vi "test_serialize_deserialize.vi"   [LabVIEW 2020, in "GPS.lvlib"]
doc: "Version 0.1"
uses:
  <vilib>/ADAS Record/CustomDataTypes/GPS/GPS.lvlib
  <vilib>/addons/_JKI Toolkits/Caraya/classes/Test/Test.lvclass
  <vilib>/addons/_JKI Toolkits/Caraya/classes/Assert/Assert.lvclass
  <vilib>/ADAS Record/CustomDataTypes/GPS/Process Data.ctl
  <vilib>/ADAS Record/CustomDataTypes/GPS/Serialize Data.vi
  <vilib>/ADAS Record/CustomDataTypes/GPS/Deserialize Data.vi
types:
  T1 = cluster{"Latitude":dbl, "Longitude":dbl, "Altitude":dbl}
  T2 = typedef "GPS.lvlib/Process Data.ctl" = cluster{"Timestamp":u64, "Antenna Connected":bool, "Satellites":u32, "Mobile Mode":bool, "Location":cluster{"Latitude":dbl, "Longitude":dbl, "Altitude":dbl}, "Velocity":cluster{"East":dbl, "North":dbl, "Up":dbl}, "GPS state":u32, "UTC Offset":i32, "UTC Offset Valid":bool}
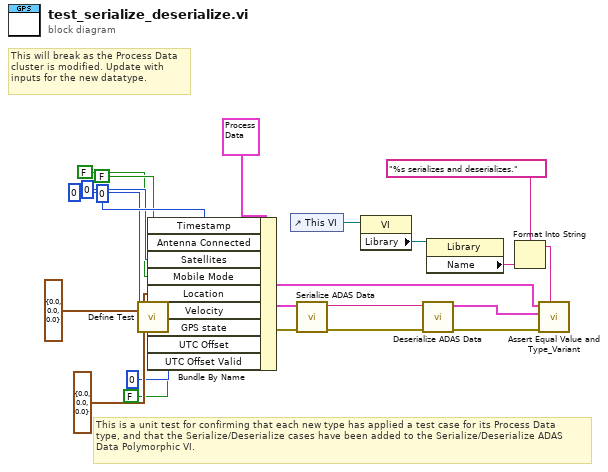
[diagram p0: block diagram]
diagram:
  # "This will break as the Process Data\ncluster is modified. Update with\ninputs for the new datatype."
  # "This is a unit test for confirming that each new type has applied a test case for its Process Data\ntype, and that the Serialize/Deserialize cases have been added to the Serialize/Deserialize ADAS\nData Polymorphic VI."
  n1 = call <vilib>:"Define Test.vi"() -> ("error out"=w16:errorcluster)  [unwired: 11 in]
  n2 = Bundle By Name "Bundle By Name"(cluster=T2 {"Timestamp"=0, "Antenna Connected"=FALSE, "Satellites"=0, "Mobile Mode"=FALSE, "Location"={"Latitude"=0.0, "Longitude"=0.0, "Altitude"=0.0}, "Velocity"={"East"=0.0, "North"=0.0, "Up"=0.0}, "GPS state"=11, "UTC Offset"=0, "UTC Offset Valid"=FALSE} ("Process Data in"), "Timestamp"=u64 0, "Antenna Connected"=FALSE, "Satellites"=u32 0, "Mobile Mode"=FALSE, "Location"=T1 {"Latitude"=0.0, "Longitude"=0.0, "Altitude"=0.0}, "Velocity"=cluster{"East":dbl, "North":dbl, "Up":dbl} {"East"=0.0, "North"=0.0, "Up"=0.0}, "GPS state"=u32 0, "UTC Offset"=0, "UTC Offset Valid"=FALSE) -> (w10:T2)
  n3 = control-ref of="This VI"() -> (w21:refnum<vi>)
  n4 = call-poly <vilib>:"Serialize ADAS Data.vi"("error in (no error)"=w16, "Process Data"=w10) -> ("error out"=w15:errorcluster, "Flat Data out"=w14:string)  [unwired: 8 in]
  n5 = property class="VI"(reference=w21) -> ("Library"=w20:refnum<vi>)  [unwired: 1 in, 2 out]
  n6 = call-poly <vilib>:"Deserialize ADAS Data.vi"("error in (no error)"=w15, "Flat Data in"=w14) -> ("error out"=w12:errorcluster, "Process Data out"=w13:T2)  [unwired: 8 in]
  n7 = property class="Library"(reference=w20) -> ("Name"=w18:string)  [unwired: 1 in, 2 out]
  n8 = Format Into String(format string="%s serializes and deserializes.", w18) -> (resulting string=w17:string)  [unwired: 2 in, 1 out]
  n9 = call <vilib>:"Assert Equal Value and Type_Variant.vi"("Label"=w17, "error in (no error)"=w12, "Y"=w13, "X"=w10) -> ()  [unwired: 7 in, 1 out]
